vi "Parse Next Single-line State.vi"(11 "States Queue":string) -> (0 "Next Single-line State":string, 3 "Remaining States Queue":string)   [LabVIEW 2014, in "Communicable State Machine.lvlib"]
uses:
  Communicable State Machine.lvlib
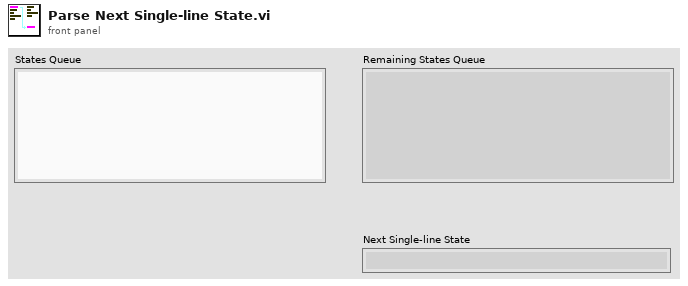
[diagram p1: front panel]
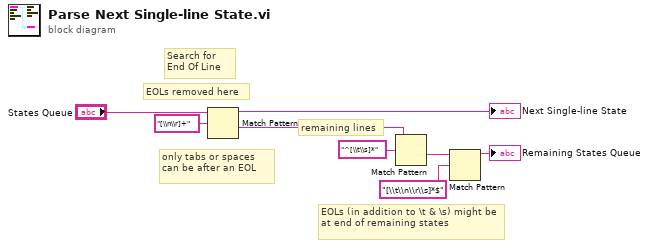
[diagram p0: block diagram]
diagram:
  # "EOLs (in addition to \\t & \\s) might be at end of remaining states"
  # "only tabs or spaces can be after an EOL"
  # "remaining lines"
  # "EOLs removed here"
  # "Search for End Of Line"
  n1 = Match Pattern(string="States Queue", regular expression="[\\n\\r]+") -> (before substring=→"Next Single-line State":string, after substring=w7:string)  [unwired: 1 in, 2 out]
  n2 = Match Pattern(string=w7, regular expression="^[\\t\\s]*") -> (after substring=w4:string)  [unwired: 1 in, 3 out]
  n3 = Match Pattern(string=w4, regular expression="[\\t\\n\\r\\s]*$") -> (before substring=→"Remaining States Queue":string)  [unwired: 1 in, 3 out]
